vi "CRYGet Frequency Curve array.vi"(8 "Additive Info":T2, 9 "Spectral Scaling":u16, 10 "Unit Info In":T4={"Y unit In"="dB", "dB ref In"=1.0, "Y unit Out"="dB", "dB ref Out"=1.0, "Y unit Curve"="dB", "dB ref Curve"=1.0, "Y data  Curve"=0, "Y data Time"=0}, 11 "Option Array In":bool[](array[boolean])) -> (1 "Display Array":T5(array[cluster]), 2 "Unit Info Out":T3[](array[typedef]), 3 "Curve Info Array Out":T1)   [LabVIEW 2013]
uses:
  Typedef Control/CRYUnit Info Cluster.ctl
  Typedef Control/CRYUnit Info Out Cluster.ctl
  Typedef Control/CRYAnalysis CurveName Cluster.ctl
  CRYMainGlobal.vi
panel:
  in  "Is Impedance?":bool
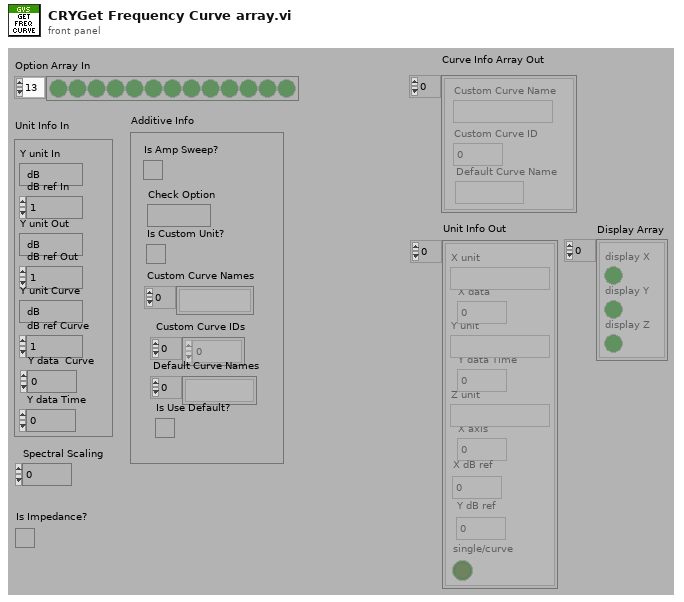
[diagram p1: front panel]
types:
  T1 = typedef "CRYAnalysis CurveName Cluster.ctl" = cluster{"Custom Curve Name":string, "Custom Curve ID":i32, "Default Curve Name":string}[]
  T2 = cluster{"Is Amp Sweep?":bool, "Check Option":string, "Is Custom Unit?":bool, "Custom Curve Names":string[], "Custom Curve IDs":i32[], "Default Curve Names":string[], "Is Use Default?":bool}
  T3 = typedef "CRYUnit Info Out Cluster.ctl" = cluster{"X unit":string, "X data":u16, "Y unit":string, "Y data Time":u16, "Z unit":string, "X axis":u16, "X dB ref":dbl, "Y dB ref":dbl, "single/curve":bool}
  T4 = typedef "CRYUnit Info Cluster.ctl" = cluster{"Y unit In":string, "dB ref In":dbl, "Y unit Out":string, "dB ref Out":dbl, "Y unit Curve":string, "dB ref Curve":dbl, "Y data  Curve":u16, "Y data Time":u16}
  T5 = cluster{"display X":bool, "display Y":bool, "display Z":bool}[]
  T6 = enum32{"English", "Chinese", "Korean", "Japanese", "Russian", "Chinese traditional"}
  T7 = cluster{"display X":bool, "display Y":bool, "display Z":bool}
  T8 = cluster{"X unit":string, "X data":u16, "Y unit Out":string, "Y data  Curve":u16, "Z unit":string, "X data":u16, "dB ref In":dbl, "dB ref Out":dbl, "display X":bool}
  T9 = cluster{"X unit":string, "X data":u16, "Y unit In":string, "Y data  Curve":u16, "Z unit":string, "X data":u16, "dB ref In":dbl, "dB ref In":dbl, "display X":bool}
  T10 = cluster{"X unit":string, "X data":u16, string, "Y data  Curve":u16, "Z unit":string, "X data":u16, "dB ref In":dbl, "dB ref In":dbl, "display X":bool}
  T11 = cluster{"X unit":string, "X data":u16, "Y unit Curve":string, "Y data  Curve":u16, "Z unit":string, "X data":u16, "dB ref In":dbl, "dB ref Curve":dbl, "display X":bool}
  T12 = cluster{"X unit":string, "X data":u16, "X unit":string, "X data":u16, "Z unit":string, "X data":u16, "dB ref In":dbl, "dB ref In":dbl, "display X":bool}
  T13 = cluster{"X unit":string, "X data":u16, "Z unit":string, "Y data  Curve":u16, "Z unit":string, "X data":u16, "dB ref In":dbl, "dB ref In":dbl, "display X":bool}
  T14 = cluster{"X unit":string, "X data":u16, "Y unit In":string, "X data":u16, "Z unit":string, "X data":u16, "dB ref In":dbl, "dB ref In":dbl, "display X":bool}
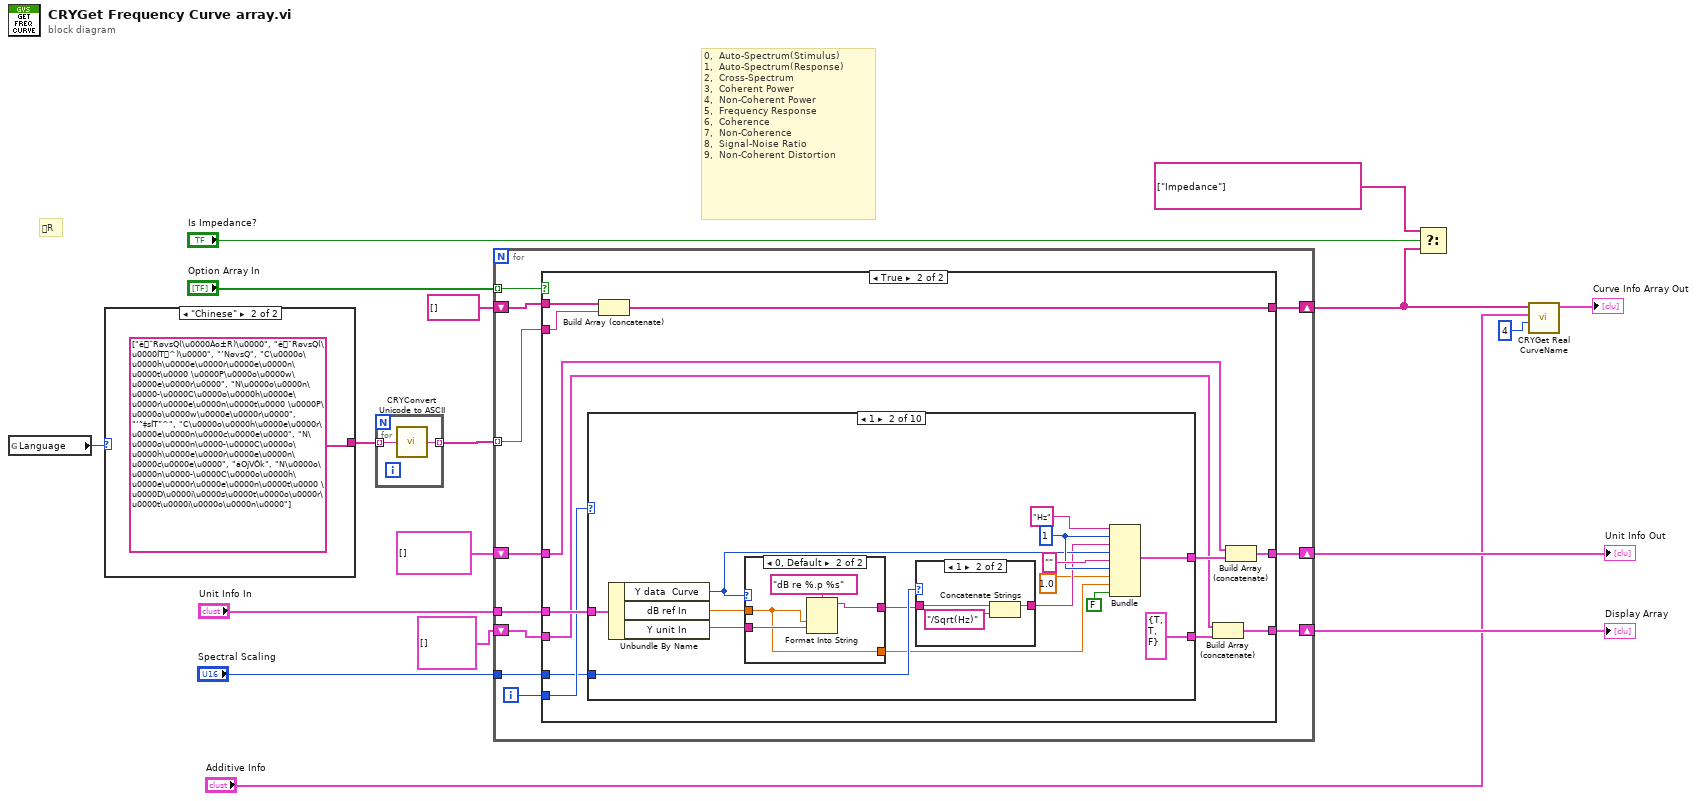
[diagram p0: block diagram]
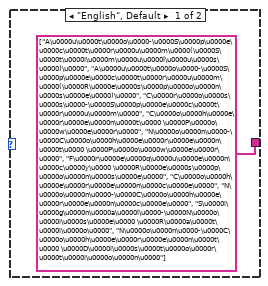
[diagram p2: hidden frame]
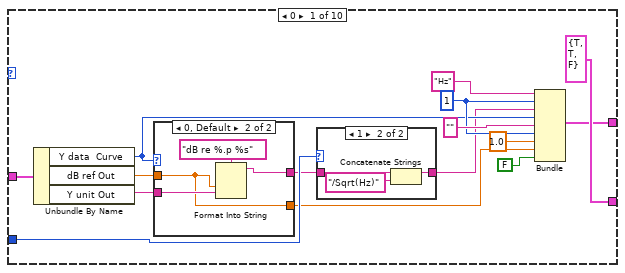
[diagram p4: hidden frame]
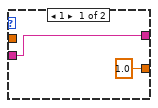
[diagram p6: hidden frame]
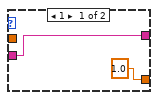
[diagram p8: hidden frame]
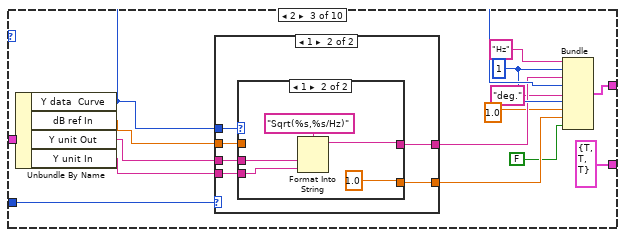
[diagram p9: hidden frame]
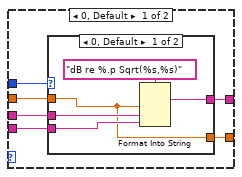
[diagram p10: hidden frame]
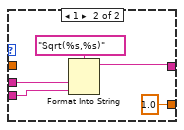
[diagram p11: hidden frame]
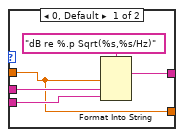
[diagram p12: hidden frame]
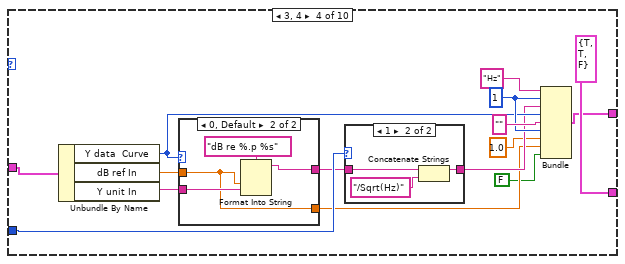
[diagram p13: hidden frame]
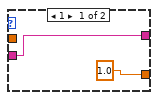
[diagram p15: hidden frame]
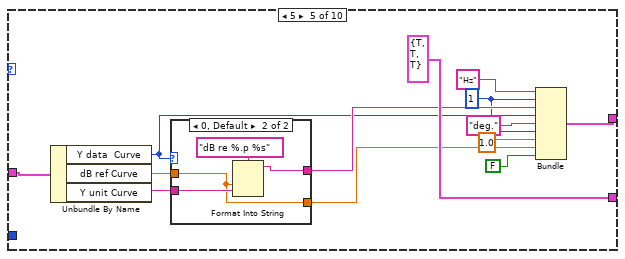
[diagram p16: hidden frame]
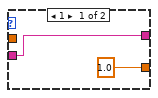
[diagram p17: hidden frame]
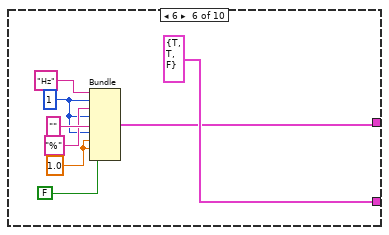
[diagram p18: hidden frame]
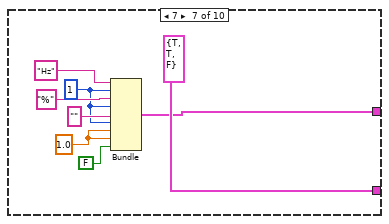
[diagram p19: hidden frame]
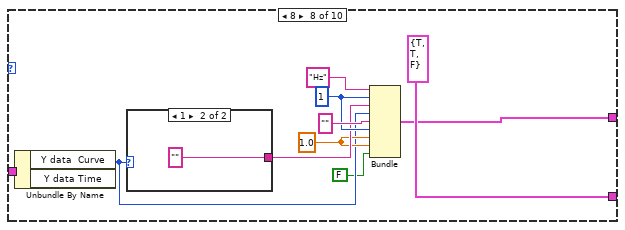
[diagram p20: hidden frame]
diagram:
  # "ꁨR"
  # "0,  Auto-Spectrum(Stimulus)\n1,  Auto-Spectrum(Response)\n2,  Cross-Spectrum\n3,  Coherent Power\n4,  Non-Coherent Power\n5,  Frequency Response\n6,  Coherence\n7,  Non-Coherence\n8,  Signal-Noise Ratio\n9,  Non-Coherent Distortion"
  n1 = global read "CRYMainGlobal.vi" "Language"() -> (w2:T6)
  n2 = case shown="\"Chinese\"" w2 {
    tunnel: [string[] ["A\u0000u\u0000t\u0000o\u0000-\u0000S\u0000p\u0000e\u0000c\u0000t\u0000r\u0000u\u0000m\u0000(\u0000S\u0000t\u0000i\u0000m\u0000u\u0000l\u0000u\u0000s\u0000)\u0000", "A\u0000u\u0000t\u0000o\u0000-\u0000S\u0000p\u0000e\u0000c\u0000t\u0000r\u0000u\u0000m\u0000(\u0000R\u0000e\u0000s\u0000p\u0000o\u0000n\u0000s\u0000e\u0000)\u0000", "C\u0000r\u0000o\u0000s\u0000s\u0000-\u0000S\u0000p\u0000e\u0000c\u0000t\u0000r\u0000u\u0000m\u0000", "C\u0000o\u0000h\u0000e\u0000r\u0000e\u0000n\u0000t\u0000 \u0000P\u0000o\u0000w\u0000e\u0000r\u0000", "N\u0000o\u0000n\u0000-\u0000C\u0000o\u0000h\u0000e\u0000r\u0000e\u0000n\u0000t\u0000 \u0000P\u0000o\u0000w\u0000e\u0000r\u0000", "F\u0000r\u0000e\u0000q\u0000u\u0000e\u0000n\u0000c\u0000y\u0000 \u0000R\u0000e\u0000s\u0000p\u0000o\u0000n\u0000s\u0000e\u0000", "C\u0000o\u0000h\u0000e\u0000r\u0000e\u0000n\u0000c\u0000e\u0000", "N\u0000o\u0000n\u0000-\u0000C\u0000o\u0000h\u0000e\u0000r\u0000e\u0000n\u0000c\u0000e\u0000", "S\u0000i\u0000g\u0000n\u0000a\u0000l\u0000-\u0000N\u0000o\u0000i\u0000s\u0000e\u0000 \u0000R\u0000a\u0000t\u0000i\u0000o\u0000", "N\u0000o\u0000n\u0000-\u0000C\u0000o\u0000h\u0000e\u0000r\u0000e\u0000n\u0000t\u0000 \u0000D\u0000i\u0000s\u0000t\u0000o\u0000r\u0000t\u0000i\u0000o\u0000n\u0000"] string[] ["ê¨RøvsQ(\u0000Ào±R)\u0000", "ê¨RøvsQ(\u0000ÍT^)\u0000", "’NøvsQ", "C\u0000o\u0000h\u0000e\u0000r\u0000e\u0000n\u0000t\u0000 \u0000P\u0000o\u0000w\u0000e\u0000r\u0000", "N\u0000o\u0000n\u0000-\u0000C\u0000o\u0000h\u0000e\u0000r\u0000e\u0000n\u0000t\u0000 \u0000P\u0000o\u0000w\u0000e\u0000r\u0000", "‘˜‡sÍT”^", "C\u0000o\u0000h\u0000e\u0000r\u0000e\u0000n\u0000c\u0000e\u0000", "N\u0000o\u0000n\u0000-\u0000C\u0000o\u0000h\u0000e\u0000r\u0000e\u0000n\u0000c\u0000e\u0000", "áOjVÔk", "N\u0000o\u0000n\u0000-\u0000C\u0000o\u0000h\u0000e\u0000r\u0000e\u0000n\u0000t\u0000 \u0000D\u0000i\u0000s\u0000t\u0000o\u0000r\u0000t\u0000i\u0000o\u0000n\u0000"]] -> w4
    frame "English", Default {
    }
    frame "Chinese" {
    }
  }
  n3 = for {
    tunnel: w4 -> [w21] mode=indexing
    tunnel: [w20] -> w3 mode=indexing
    n4 = call "CRYConvert Unicode to ASCII.vi"("Unicode"=w21) -> ("ASCII"=w20:string)  [unwired: 4 in]
  }
  n5 = for {
    tunnel: w3 -> [w30] mode=indexing
    tunnel: "Option Array In" -> [w32] mode=indexing
    shift-right: [w29] -> w1
    shift-left: string[] [] ("Array") -> [w31]
    shift-right: [w26] -> w10
    shift-left: T3[] [] ("Unit Info Out") -> [w24]
    tunnel: "Unit Info In" -> [w27]
    shift-right: [w25] -> w14
    shift-left: T5 [] -> [w23]
    tunnel: "Spectral Scaling" -> [w22]
    i -> [w28]
    n6 = case shown="True" w32 {
      tunnel: w31 -> [w35 w47]
      tunnel: w30 -> [_ w46]
      tunnel: [w35 w45] -> w29
      tunnel: w28 -> [_ w37]
      tunnel: w27 -> [_ w44]
      tunnel: [w34 w42] -> w26
      tunnel: [w33 w40] -> w25
      tunnel: w24 -> [w34 w39]
      tunnel: w23 -> [w33 w38]
      tunnel: w22 -> [_ w36]
      frame False {
      }
      frame True {
        n7 = case shown="1" w37 {
          tunnel: [T7 {"display X"=TRUE, "display Y"=TRUE, "display Z"=FALSE} T7 {"display X"=TRUE, "display Y"=TRUE, "display Z"=FALSE} T7 {"display X"=TRUE, "display Y"=TRUE, "display Z"=TRUE} T7 {"display X"=TRUE, "display Y"=TRUE, "display Z"=FALSE} T7 {"display X"=TRUE, "display Y"=TRUE, "display Z"=TRUE} T7 {"display X"=TRUE, "display Y"=TRUE, "display Z"=FALSE} T7 {"display X"=TRUE, "display Y"=TRUE, "display Z"=FALSE} T7 {"display X"=TRUE, "display Y"=TRUE, "display Z"=FALSE} T7 {"display X"=TRUE, "display Y"=TRUE, "display Z"=FALSE} _] -> w41
          tunnel: w44 -> [w54 w79 w102 w151 w174 _ _ w209 w224 _]
          tunnel: [w55 w80 w104 w152 w173 w191 w199 w210 w223 _] -> w43
          tunnel: w36 -> [w53 w78 w103 w150 _ _ _ _ w221 _]
          frame 0 {
            w59 = u16 1 ("X data")
            n8 = Unbundle By Name(w54) -> ("Y data  Curve"=w56:u16, "dB ref Out"=w58:dbl, "Y unit Out"=w57:string)
            n9 = case shown="0, Default" w56 {
              tunnel: [w68 w70] -> w52
              tunnel: w58 -> [_ w69]
              tunnel: w57 -> [w68 w71]
              tunnel: [1.0 ("dB ref Out") w69] -> w50
              frame 1 {
              }
              frame 0, Default {
                n10 = Format Into String(format string="dB re %.p %s", w69, w71) -> (resulting string=w70:string)  [unwired: 2 in, 1 out]
              }
            }
            n11 = case shown="1" w53 {
              tunnel: w52 -> [w63 w66]
              tunnel: [w63 w65] -> w51
              frame 0, Default {
              }
              frame 1 {
                n12 = Concatenate Strings(w66, "/Sqrt(Hz)" ("string")) -> (w65:string)
              }
            }
            n13 = Bundle("X unit"="Hz", "X data"=w59, "Y unit Out"=w51, "Y data  Curve"=w56, "Z unit"="", "X data"=w59, "dB ref In"=1.0, "dB ref Out"=w50, "display X"=FALSE) -> (w55:T8)  [unwired: 1 in]
          }
          frame 1 {
            w84 = u16 1 ("X data")
            n14 = Unbundle By Name(w79) -> ("Y data  Curve"=w81:u16, "dB ref In"=w83:dbl, "Y unit In"=w82:string)
            n15 = case shown="0, Default" w81 {
              tunnel: [w93 w95] -> w77
              tunnel: w83 -> [_ w94]
              tunnel: w82 -> [w93 w96]
              tunnel: [1.0 ("dB ref In") w94] -> w75
              frame 1 {
              }
              frame 0, Default {
                n16 = Format Into String(format string="dB re %.p %s", w94, w96) -> (resulting string=w95:string)  [unwired: 2 in, 1 out]
              }
            }
            n17 = case shown="1" w78 {
              tunnel: w77 -> [w88 w91]
              tunnel: [w88 w90] -> w76
              frame 0, Default {
              }
              frame 1 {
                n18 = Concatenate Strings(w91, "/Sqrt(Hz)" ("string")) -> (w90:string)
              }
            }
            n19 = Bundle("X unit"="Hz", "X data"=w84, "Y unit In"=w76, "Y data  Curve"=w81, "Z unit"="", "X data"=w84, "dB ref In"=1.0, "dB ref In"=w75, "display X"=FALSE) -> (w80:T9)  [unwired: 1 in]
          }
          frame 2 {
            w109 = u16 1 ("X data")
            n20 = Unbundle By Name(w102) -> ("Y data  Curve"=w111:u16, "dB ref In"=w101:dbl, "Y unit Out"=w110:string, "Y unit In"=w105:string)
            n21 = case shown="1" w103 {
              tunnel: w111 -> [w118 w134]
              tunnel: w110 -> [w117 w133]
              tunnel: w101 -> [w116 w132]
              tunnel: [w115 w131] -> w108
              tunnel: w105 -> [w114 w130]
              tunnel: [w113 w129] -> w100
              frame 0, Default {
                n22 = case shown="0, Default" w118 {
                  tunnel: [w122 w125] -> w115
                  tunnel: w116 -> [w119 _]
                  tunnel: w117 -> [w121 w127]
                  tunnel: w114 -> [w120 w126]
                  tunnel: [w119 1.0 ("dB ref In")] -> w113
                  frame 0, Default {
                    n23 = Format Into String(format string="dB re %.p Sqrt(%s,%s)", w119, w121, w120) -> (resulting string=w122:string)  [unwired: 2 in, 1 out]
                  }
                  frame 1 {
                    n24 = Format Into String(format string="Sqrt(%s,%s)", w127, w126) -> (resulting string=w125:string)  [unwired: 2 in, 1 out]
                  }
                }
              }
              frame 1 {
                n25 = case shown="1" w134 {
                  tunnel: [w138 w141] -> w131
                  tunnel: w132 -> [w135 _]
                  tunnel: w133 -> [w137 w143]
                  tunnel: w130 -> [w136 w142]
                  tunnel: [w135 1.0 ("dB ref In")] -> w129
                  frame 0, Default {
                    n26 = Format Into String(format string="dB re %.p Sqrt(%s,%s/Hz)", w135, w137, w136) -> (resulting string=w138:string)  [unwired: 2 in, 1 out]
                  }
                  frame 1 {
                    n27 = Format Into String(format string="Sqrt(%s,%s/Hz)", w143, w142) -> (resulting string=w141:string)  [unwired: 2 in, 1 out]
                  }
                }
              }
            }
            n28 = Bundle("X unit"="Hz", "X data"=w109, w108, "Y data  Curve"=w111, "Z unit"="deg.", "X data"=w109, "dB ref In"=1.0, "dB ref In"=w100, "display X"=FALSE) -> (w104:T10)  [unwired: 1 in]
          }
          frame 3, 4 {
            w156 = u16 1 ("X data")
            n29 = Unbundle By Name(w151) -> ("Y data  Curve"=w153:u16, "dB ref In"=w155:dbl, "Y unit In"=w154:string)
            n30 = case shown="0, Default" w153 {
              tunnel: [w165 w167] -> w149
              tunnel: w155 -> [_ w166]
              tunnel: w154 -> [w165 w168]
              tunnel: [1.0 ("dB ref In") w166] -> w147
              frame 1 {
              }
              frame 0, Default {
                n31 = Format Into String(format string="dB re %.p %s", w166, w168) -> (resulting string=w167:string)  [unwired: 2 in, 1 out]
              }
            }
            n32 = case shown="1" w150 {
              tunnel: w149 -> [w160 w163]
              tunnel: [w160 w162] -> w148
              frame 0, Default {
              }
              frame 1 {
                n33 = Concatenate Strings(w163, "/Sqrt(Hz)" ("string")) -> (w162:string)
              }
            }
            n34 = Bundle("X unit"="Hz", "X data"=w156, "Y unit In"=w148, "Y data  Curve"=w153, "Z unit"="", "X data"=w156, "dB ref In"=1.0, "dB ref In"=w147, "display X"=FALSE) -> (w152:T9)  [unwired: 1 in]
          }
          frame 5 {
            w178 = u16 1 ("X data")
            n35 = Unbundle By Name(w174) -> ("Y data  Curve"=w175:u16, "dB ref Curve"=w177:dbl, "Y unit Curve"=w176:string)
            n36 = case shown="0, Default" w175 {
              tunnel: [w184 w186] -> w179
              tunnel: w177 -> [_ w185]
              tunnel: w176 -> [w184 w187]
              tunnel: [1.0 ("dB ref In") w185] -> w172
              frame 1 {
              }
              frame 0, Default {
                n37 = Format Into String(format string="dB re %.p %s", w185, w187) -> (resulting string=w186:string)  [unwired: 2 in, 1 out]
              }
            }
            n38 = Bundle("X unit"="Hz", "X data"=w178, "Y unit Curve"=w179, "Y data  Curve"=w175, "Z unit"="deg.", "X data"=w178, "dB ref In"=1.0, "dB ref Curve"=w172, "display X"=FALSE) -> (w173:T11)  [unwired: 1 in]
          }
          frame 6 {
            w190 = 1.0 ("dB ref In")
            w192 = u16 1 ("X data")
            n39 = Bundle("X unit"="Hz", "X data"=w192, "X unit"="%", "X data"=w192, "Z unit"="", "X data"=w192, "dB ref In"=w190, "dB ref In"=w190, "display X"=FALSE) -> (w191:T12)  [unwired: 1 in]
          }
          frame 7 {
            w198 = 1.0 ("dB ref In")
            w200 = u16 1 ("X data")
            n40 = Bundle("X unit"="Hz", "X data"=w200, "X unit"="%", "X data"=w200, "Z unit"="", "X data"=w200, "dB ref In"=w198, "dB ref In"=w198, "display X"=FALSE) -> (w199:T12)  [unwired: 1 in]
          }
          frame 8 {
            w207 = 1.0 ("dB ref In")
            w211 = u16 1 ("X data")
            n41 = Unbundle By Name(w209) -> ("Y data  Curve"=w206:u16)  [unwired: 1 out]
            n42 = case shown="1" w206 {
              tunnel: ["dB re 1" ("X unit") "" ("Z unit")] -> w208
              frame 0, Default {
              }
              frame 1 {
              }
            }
            n43 = Bundle("X unit"="Hz", "X data"=w211, "Z unit"=w208, "Y data  Curve"=w206, "Z unit"="", "X data"=w211, "dB ref In"=w207, "dB ref In"=w207, "display X"=FALSE) -> (w210:T13)  [unwired: 1 in]
          }
          frame 9 {
            w222 = 1.0 ("dB ref In")
            w218 = u16 1 ("X data")
            n44 = Unbundle By Name(w224) -> ()  [unwired: 3 out]
            n45 = case shown="0, Default" w221 {
              tunnel: "%" ("Y unit In") -> [w228 w231]
              tunnel: [w228 w230] -> w220
              frame 0, Default {
              }
              frame 1 {
                n46 = Concatenate Strings(w231, "/Sqrt(Hz)" ("string")) -> (w230:string)
              }
            }
            n47 = Bundle("X unit"="Hz", "X data"=w218, "Y unit In"=w220, "X data"=w218, "Z unit"="", "X data"=w218, "dB ref In"=w222, "dB ref In"=w222, "display X"=FALSE) -> (w223:T14)  [unwired: 1 in]
          }
          frame Default {
          }
        }
        n48 = Build Array (concatenate)(w47, w46) -> (w45:string[])
        n49 = Build Array (concatenate)(w38, w41) -> (w40:T5)
        n50 = Build Array (concatenate)(w39, w43) -> (w42:T3[])
      }
    }
  }
  "Display Array" <- w14
  "Unit Info Out" <- w10
  n51 = Select(t=string[] ["Impedance"], s="Is Impedance?", f=w1) -> ()  [unwired: 1 out]
  n52 = call "CRYGet Real CurveName.vi"("Key No"=4, "Additive Info"="Additive Info", "CurveArrayByType"=w1) -> ("Curve Info Array Out"=→"Curve Info Array Out":T1)  [unwired: 8 in]
